vi "Day 4.2 - Find last to win.vi"(9 "bingo cards":i32[][][](array[numeric]), 11 "bingo calls":i32[](array[numeric])) -> (3 "output":u32)   [LabVIEW 2021]
panel:
  out "Winning Card":i32
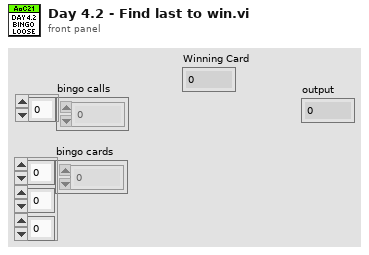
[diagram p1: front panel]
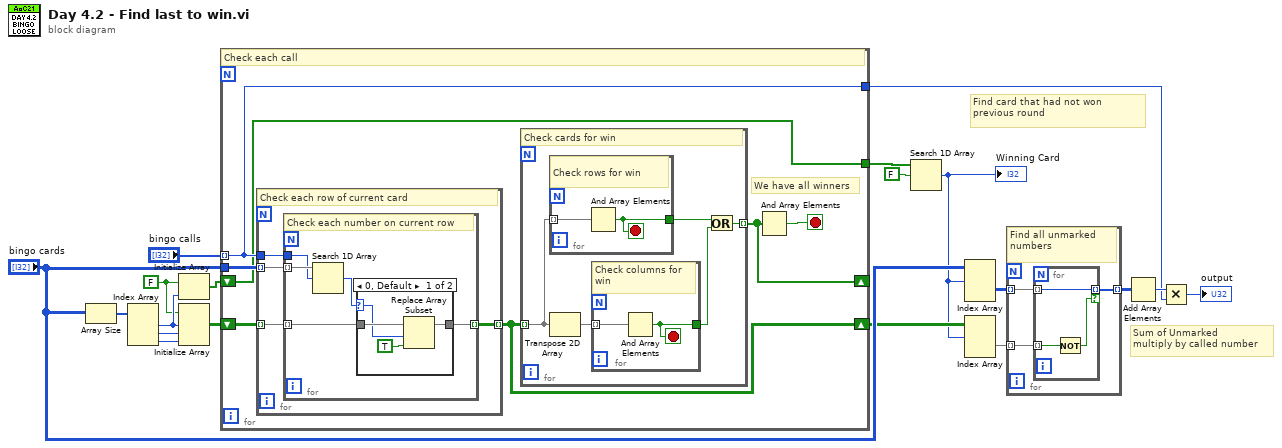
[diagram p0: block diagram]
diagram:
  w12 = FALSE
  # "Find card that had not won previous round"
  # "Sum of Unmarked\nmultiply by called number"
  n1 = Array Size(array="bingo cards") -> (size(s)=w18:i32[])
  n2 = Index Array(array=w18) -> (element #1=w13:i32, element #2=w17:i32, element #3=w16:i32)  [unwired: 3 in]
  n3 = Initialize Array(w12, w13) -> (w14:bool[])
  n4 = Initialize Array(w12, w13, w17, w16) -> (w15:bool[][][])
  n5 = for {
    tunnel: "bingo calls" -> [w21] mode=indexing
    shift-right: [w25] -> w9
    shift-left: w15 -> [w26]
    shift-right: [w23] -> _
    shift-left: w14 -> [w20]
    tunnel: "bingo cards" -> [w24]
    tunnel: [w21] -> w2
    tunnel: [w20] -> w1
    stop <- w22 stop-if-true
    # "We have all winners"
    # "Check each call"
    n6 = for {
      tunnel: w24 -> [w39] mode=indexing
      tunnel: w26 -> [w37] mode=indexing
      tunnel: w21 -> [w38]
      tunnel: [w36] -> w25 mode=indexing
      # "Check each row of current card"
      n7 = for {
        tunnel: w39 -> [w44] mode=indexing
        tunnel: w38 -> [w43]
        tunnel: w37 -> [w41] mode=indexing
        tunnel: [w40] -> w36 mode=indexing
        # "Check each number on current row"
        n8 = Search 1D Array(1D array=w44, element=w43) -> (index of element=w42:i32)  [unwired: 1 in]
        n9 = case shown="0, Default" w42 {
          selector: w42 -> [w47 _]
          tunnel: [w45 w49] -> w40
          tunnel: w41 -> [w48 w49]
          frame 0, Default {
            n10 = Replace Array Subset(array=w48, new element=TRUE ("new element/subarray"), index=w47) -> (w45:bool[])
          }
          frame -1 {
          }
        }
      }
    }
    n11 = for {
      tunnel: w25 -> [w31] mode=indexing
      tunnel: [w27] -> w23 mode=indexing
      # "Check cards for win"
      n12 = for {
        tunnel: w31 -> [w35] mode=indexing
        tunnel: [w34] -> w29
        stop <- w34 stop-if-true
        # "Check rows for win"
        n13 = And Array Elements(Boolean array=w35) -> (logical AND=w34:bool)
      }
      n14 = Transpose 2D Array(2D array=w31) -> (transposed array=w30:bool[][])
      n15 = for {
        tunnel: w30 -> [w33] mode=indexing
        tunnel: [w32] -> w28
        stop <- w32 stop-if-true
        # "Check columns for win"
        n16 = And Array Elements(Boolean array=w33) -> (logical AND=w32:bool)
      }
      n17 = Or(x=w29, y=w28) -> (x .or. y?=w27:bool)
    }
    n18 = And Array Elements(Boolean array=w23) -> (logical AND=w22:bool)
  }
  n19 = Search 1D Array(1D array=w1, element=FALSE) -> (index of element=w8:i32)  [unwired: 1 in]
  "Winning Card" <- w8
  n20 = Index Array(array="bingo cards", index (dim 0)=w8) -> (element=w7:i32[][])  [unwired: 2 in]
  n21 = Index Array(array=w9, index (dim 0)=w8) -> (element=w6:bool[][])  [unwired: 2 in]
  n22 = for {
    tunnel: w7 -> [w52] mode=indexing
    tunnel: w6 -> [w51] mode=indexing
    tunnel: [w50] -> w5 mode=indexing
    # "Find all unmarked numbers"
    n23 = for {
      tunnel: w52 -> [w55] mode=indexing
      tunnel: w51 -> [w54] mode=indexing
      tunnel: [w55] -> w50 mode=indexing if=w53
      n24 = Not(x=w54) -> (.not. x?=w53:bool)
    }
  }
  n25 = Add Array Elements(numeric array=w5) -> (sum=w4:i32)
  n26 = Multiply(x=w4, y=w2) -> (x*y=→"output":i32)
